vi "Fire Stop Event.vi"(8 "error in (no error)":errorcluster, 11 "Stop Event in":refnum<user-event>) -> (0 "error out":errorcluster, 3 "Stop Event out":refnum<user-event>)   [LabVIEW 2016, in "Stop Event.lvlib"]
uses:
  Stop Event.lvlib
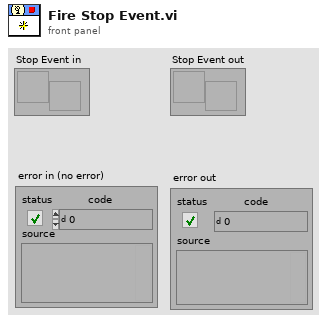
[diagram p1: front panel]
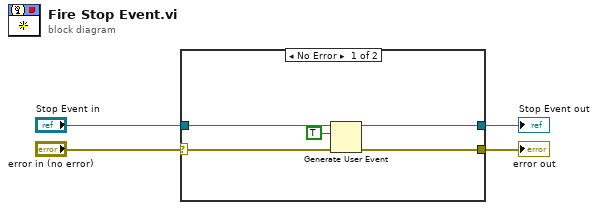
[diagram p0: block diagram]
diagram:
  n1 = case shown="No Error" "error in (no error)" {
    selector: "error in (no error)" -> [w9 w11]
    tunnel: [w8 w11] -> w3
    tunnel: [w7 w10] -> w2
    tunnel: "Stop Event in" -> [w6 w10]
    frame No Error {
      n2 = Generate User Event(user event=w6, event data cluster=TRUE ("event data"), error in=w9) -> (user event out=w7:refnum<user-event>, error out=w8:errorcluster)  [unwired: 1 in]
    }
    frame Error {
    }
  }
  "error out" <- w3
  "Stop Event out" <- w2
